vi "Main.vi"() -> ()   [LabVIEW 2020]
uses:
  <vilib>/SAPHIR/GDataBase for MySQL(tm)/MySQL/MySQLConnector.lvclass/MySQLConnector.ctl
  <vilib>/SAPHIR/GDataBase for MySQL(tm)/NetworkStream/MySQLNetworkStream.lvclass/MySQLNetworkStream.ctl
  <vilib>/SAPHIR/GDataBase for MySQL(tm)/NetworkStream/public/SendCommand.vi
  <vilib>/SAPHIR/GDataBase for MySQL(tm)/NetworkStream/public/locker/AcquireLocker.vi
  <vilib>/SAPHIR/GDataBase for MySQL(tm)/NetworkStream/public/locker/ReleaseLocker.vi
  <vilib>/SAPHIR/GDataBase for MySQL(tm)/NetworkStream/public/WritePacket.vi
  <vilib>/Utility/semaphor.llb/Acquire Semaphore.vi
  <vilib>/SAPHIR/GDataBase for MySQL(tm)/NetworkStream/public/ReadResultPacket.vi
  <vilib>/Utility/semaphor.llb/Release Semaphore.vi
  <vilib>/Instr/_visa.llb/VISA Configure Serial Port (Instr).vi
  <vilib>/SAPHIR/GDataBase for MySQL(tm)/MySQL/MySQLConnector.lvclass
panel:
  in  "Stop":bool
  in  "Tab Control":enum32{"Dashboard", "Config"}(tab)
  out "Abanico":bool
  out "Extractor":bool
  out "Presencia de Gas":bool
  out "Alarma de Temperatura":bool
  out "Propano":dbl(slide) scale=0.0..40.0
  out "CO":dbl(slide) scale=0.0..100.0
  out "LPG":dbl(slide) scale=0.0..80.0
  out "Alcohol":dbl(slide) scale=0.0..30.0
  out "H2":dbl(slide) scale=0.0..50.0
  out "Humedad Relativa":dbl(graph)
  out "Temperatura (Celsius)":dbl(graph)
  out "Propano":dbl
  out "CO":dbl
  out "Alcohol":dbl
  out "LPG":dbl
  out "H2":dbl
  out "Hum %":dbl
  out "Temp C":dbl
  out "Fecha":string
  in  "Base de Datos":string
  in  "Password":string
  in  "Usuario":string
  in  "MySQL Server (IP)":string
  in  "Propano":dbl(slide) scale=0.0..100.0
  in  "Alcohol":dbl(slide) scale=0.0..100.0
  in  "CO":dbl(slide) scale=0.0..100.0
  in  "LPG":dbl(slide) scale=0.0..100.0
  in  "H2":dbl(slide) scale=0.0..100.0
  in  "Rango de Temperatura Adecuada":cluster{"Numeric":dbl, "Numeric":dbl}(slide)={"Numeric"=0.0, "Numeric"=6.538461538461539} scale=0.0..50.0
  in  "Puerto Serial":refnum<visa-resource-name>="COM4"
  # "Arduino"
  # "Set Points"
  # "Base de Datos"
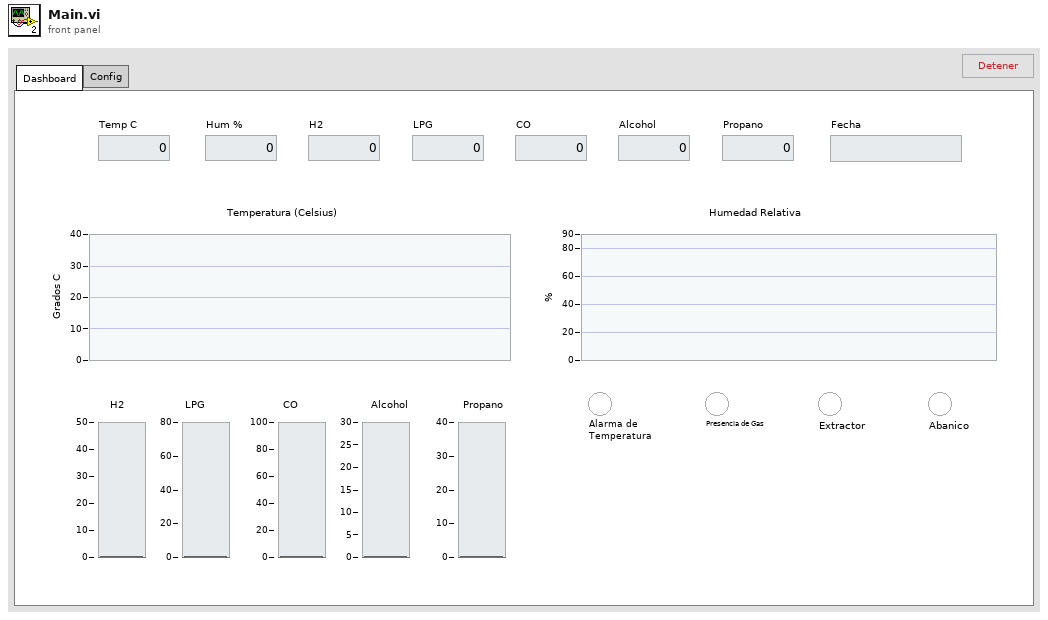
[diagram p1: front panel]
types:
  T1 = cluster{"Usuario":string, "Password":string, "Base de Datos":string}
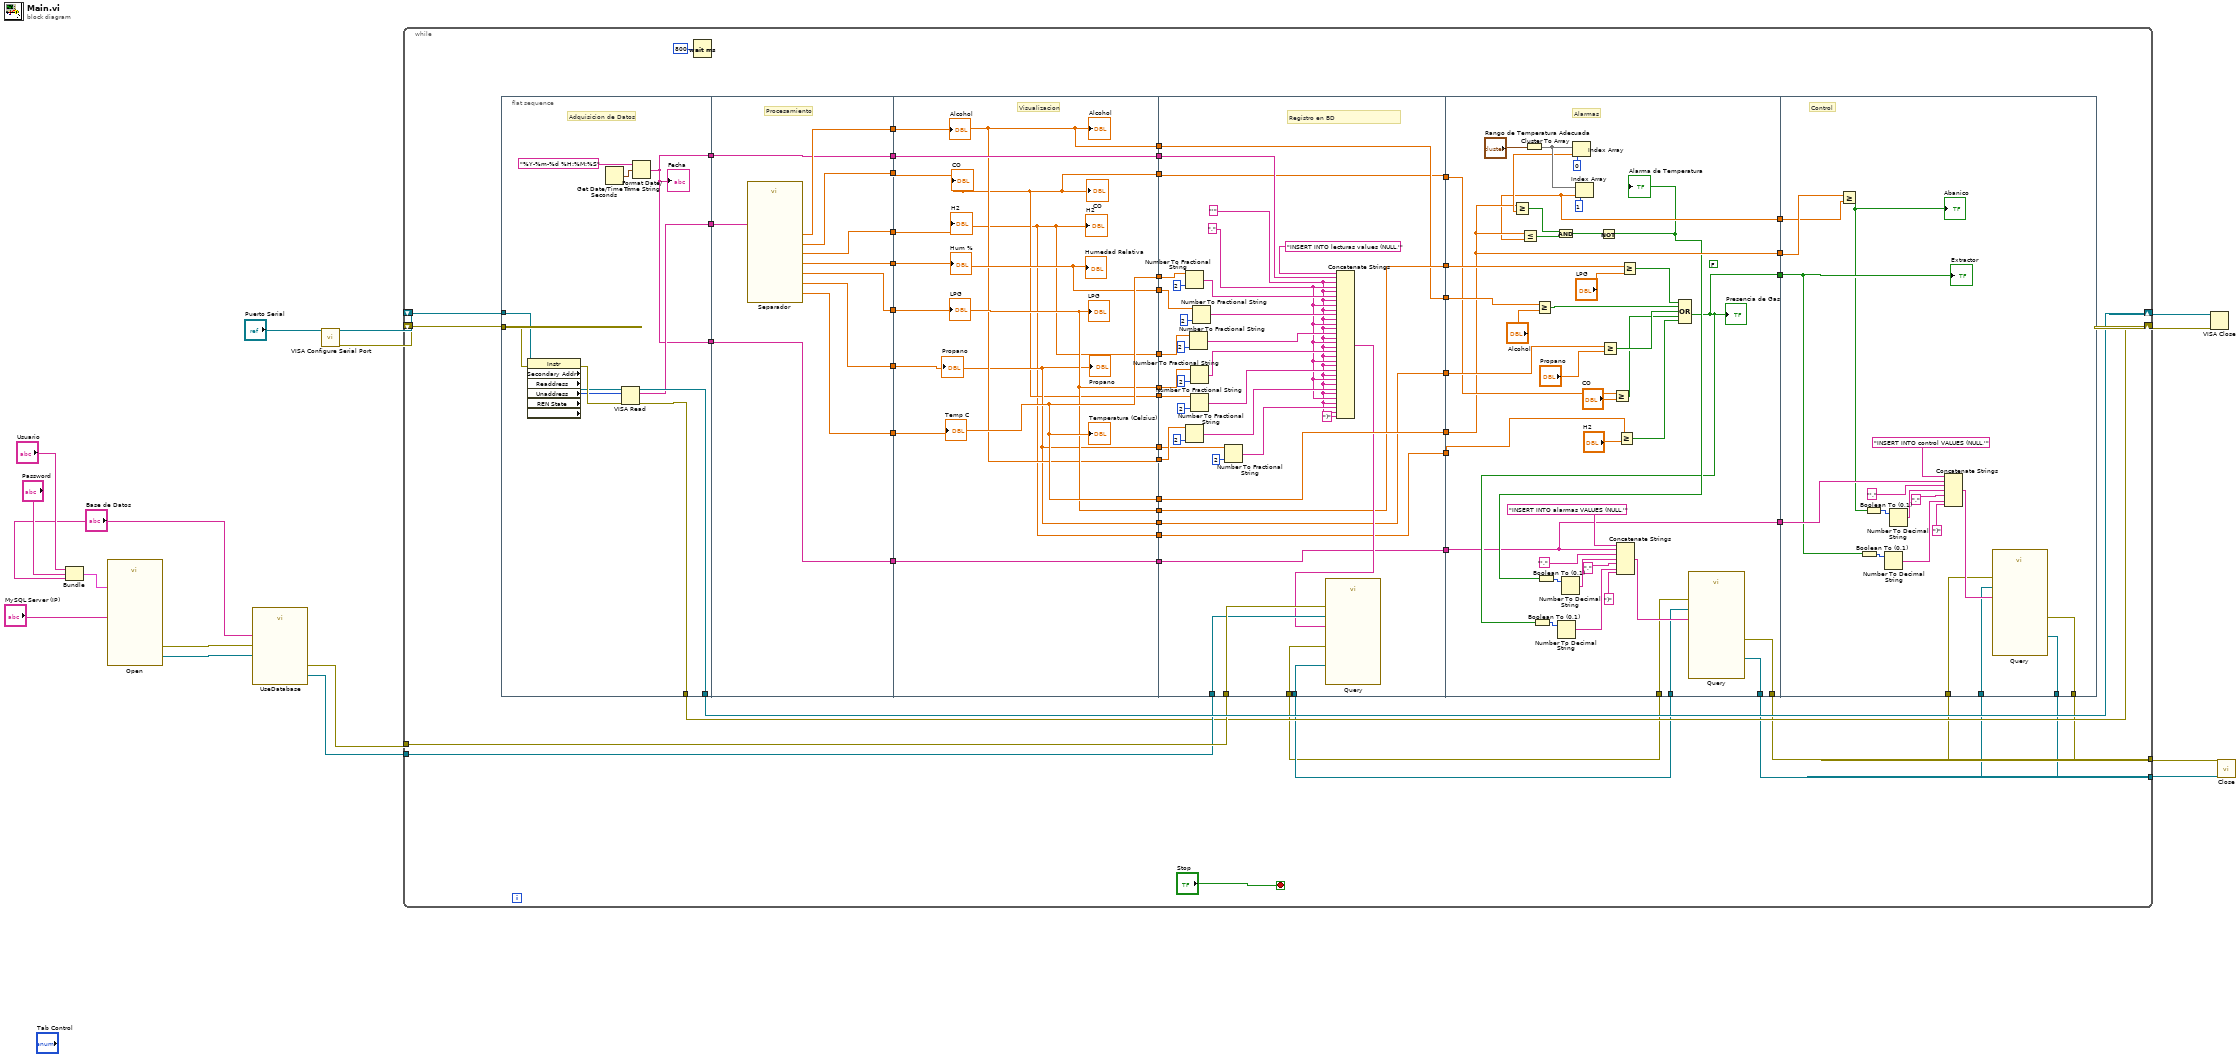
[diagram p0: block diagram]
diagram:
  n1 = Bundle("Usuario"="Usuario", "Password"="Password", "Base de Datos"="Base de Datos") -> (w1:T1)  [unwired: 1 in]
  n2 = call <vilib>:"Open.vi"("clientAuthentication"=w1, "host"="MySQL Server (IP)") -> ("error out"=w15:errorcluster, "MySQL out"=w14:refnum<class "MySQLConnector.lvclass">)  [unwired: 8 in]
  n3 = call <vilib>:"UseDatabase.vi"("error in (no error)"=w15, "databaseName"="Base de Datos", "MySQL in"=w14) -> ("error out"=w7:errorcluster, "MySQL out"=w6:refnum<class "MySQLConnector.lvclass">)  [unwired: 7 in]
  n4 = call-poly "VISA Configure Serial Port"("VISA resource name"="Puerto Serial") -> ("VISA resource name out"=w9:refnum<visa-resource-name>, "error out"=w8:errorcluster)  [unwired: 13 in]
  n5 = while {
    shift-right: [w64] -> w11
    shift-left: w9 -> [w66]
    shift-right: [w24] -> w10
    shift-left: w8 -> [w65]
    tunnel: w7 -> [w53]
    tunnel: w6 -> [w52]
    tunnel: [w19] -> w12
    tunnel: [w17] -> w13
    stop <- "Stop" stop-if-true
    n6 = flat-sequence {
      tunnel: w66 -> [w79]
      tunnel: w65 -> [w78]
      tunnel: [w74] -> w24
      tunnel: [w73] -> w64
      tunnel: [w72] -> w56
      tunnel: [w69] -> w49
      tunnel: [w69] -> w28
      tunnel: [w89] -> w63
      tunnel: [w88] -> w62
      tunnel: [w87] -> w61
      tunnel: [w86] -> w60
      tunnel: [w85] -> w59
      tunnel: [w84] -> w58
      tunnel: [w83] -> w57
      tunnel: w56 -> [w82]
      tunnel: [w81] -> w50
      tunnel: w49 -> [w81]
      tunnel: w28 -> [w80]
      tunnel: [w80] -> w27
      tunnel: w63 -> [w94]
      tunnel: w62 -> [w92]
      tunnel: w61 -> [w91]
      tunnel: w60 -> [w96]
      tunnel: w59 -> [w95]
      tunnel: w58 -> [w93]
      tunnel: w57 -> [w97]
      tunnel: [w97] -> w55
      tunnel: [w98] -> w51
      tunnel: w50 -> [w98]
      tunnel: [w97] -> w48
      tunnel: [w96] -> w47
      tunnel: [w91] -> w46
      tunnel: [w95] -> w45
      tunnel: [w92] -> w44
      tunnel: [w94] -> w43
      tunnel: [w93] -> w42
      tunnel: [w95] -> w41
      tunnel: [w94] -> w39
      tunnel: [w93] -> w37
      tunnel: [w92] -> w34
      tunnel: [w91] -> w33
      tunnel: w27 -> [w90]
      tunnel: [w90] -> w26
      tunnel: w55 -> [w136]
      tunnel: [w136] -> w54
      tunnel: w53 -> [w135]
      tunnel: w52 -> [w134]
      tunnel: [w133] -> w22
      tunnel: [w132] -> w23
      tunnel: w51 -> [w130]
      tunnel: w48 -> [w129]
      tunnel: w47 -> [w127]
      tunnel: w46 -> [w125]
      tunnel: w45 -> [w120]
      tunnel: w44 -> [w116]
      tunnel: w43 -> [w112]
      tunnel: w42 -> [w106]
      tunnel: w41 -> [w104]
      tunnel: [w104] -> w40
      tunnel: w39 -> [w103]
      tunnel: [w103] -> w38
      tunnel: w37 -> [w102]
      tunnel: [w102] -> w36
      tunnel: [w101] -> w35
      tunnel: w34 -> [w101]
      tunnel: w33 -> [w100]
      tunnel: [w100] -> w32
      tunnel: w26 -> [w99]
      tunnel: [w99] -> w25
      tunnel: w54 -> [w154]
      tunnel: w40 -> [w165]
      tunnel: w38 -> [w164]
      tunnel: w36 -> [w163]
      tunnel: w35 -> [w162]
      tunnel: w32 -> [w161]
      tunnel: [w142] -> w31
      tunnel: [w154] -> w30
      tunnel: [w153] -> w29
      tunnel: w25 -> [w137]
      tunnel: w23 -> [w146]
      tunnel: w22 -> [w145]
      tunnel: [w144] -> w18
      tunnel: [w143] -> w20
      tunnel: [w137] -> w21
      tunnel: w31 -> [w183]
      tunnel: w30 -> [w195]
      tunnel: w29 -> [w194]
      tunnel: w21 -> [w184]
      tunnel: w20 -> [w181]
      tunnel: w18 -> [w180]
      tunnel: [w179] -> w19
      tunnel: [w178] -> w17
      frame #0 {
        # "Adquisicion de Datos"
        n7 = property class="Instr" props=["Secondary Addr", "Readdress", "Unaddress", "REN State", "Serial Settings:Number of Bytes at Serial Port"](reference=w79, error in=w78) -> (reference out=w75:refnum<visa-resource-name>, error out=w77:errorcluster, "Serial Settings:Number of Bytes at Serial Port"=w76:u32)  [unwired: 4 out]
        n8 = Get Date/Time In Seconds() -> (seconds since 1Jan1904=w71:timestamp)
        n9 = VISA Read(VISA resource name=w75, byte count=w76, error in (no error)=w77) -> (VISA resource name out=w73:refnum<visa-resource-name>, read buffer=w72:string, error out=w74:errorcluster)  [unwired: 1 out]
        n10 = Format Date/Time String(time format string (%c)="%Y-%m-%d %H:%M:%S", seconds (now)=w71) -> (date/time string=w69:string)  [unwired: 1 in]
        "Fecha" <- w69
      }
      frame #1 {
        # "Procesamiento"
        n11 = call "Separador.vi"("Lectura del puerto Serial"=w82) -> ("Propano"=w84:dbl, "ALcohol"=w89:dbl, "CO"=w88:dbl, "LPG"=w85:dbl, "H2"=w87:dbl, "Humedad"=w86:dbl, "Temperatura"=w83:dbl)
      }
      frame #2 {
        # "Visualizacion"
        "Alcohol" <- w94
        "CO" <- w92
        "H2" <- w91
        "LPG" <- w95
        "Propano" <- w93
        "Temp C" <- w97
        "Hum %" <- w96
        "Temperatura (Celsius)" <- w97
        "Humedad Relativa" <- w96
        "H2" <- w91
        "Alcohol" <- w94
        "Propano" <- w93
        "CO" <- w92
        "LPG" <- w95
      }
      frame #3 {
        w110 = ","
        w108 = "'"
        # "Registro en BD"
        n12 = Number To Fractional String(number=w129, precision (6)=i16 2) -> (F-format string=w128:string)  [unwired: 2 in]
        n13 = Number To Fractional String(number=w112, precision (6)=i16 2) -> (F-format string=w111:string)  [unwired: 2 in]
        n14 = Number To Fractional String(number=w125, precision (6)=i16 2) -> (F-format string=w124:string)  [unwired: 2 in]
        n15 = Number To Fractional String(number=w120, precision (6)=i16 2) -> (F-format string=w118:string)  [unwired: 2 in]
        n16 = Number To Fractional String(number=w116, precision (6)=i16 2) -> (F-format string=w117:string)  [unwired: 2 in]
        n17 = Number To Fractional String(number=w127, precision (6)=i16 2) -> (F-format string=w126:string)  [unwired: 2 in]
        n18 = Number To Fractional String(number=w106, precision (6)=i16 2) -> (F-format string=w109:string)  [unwired: 2 in]
        n19 = Concatenate Strings("INSERT INTO lecturas values (NULL,'" ("string"), w130, w108, w110, w108, w128, w108, w110, w108, w126, w108, w110, w108, w124, w108, w110, w108, w118, w108, w110, w108, w117, w108, w110, w108, w111, w108, w110, w108, w109, w108, ")" ("string")) -> (w105:string)
        n20 = call <vilib>:"Query.vi"("error in (no error)"=w135, "query"=w105, "MySQL in"=w134) -> ("error out"=w133:errorcluster, "MySQL out"=w132:refnum<class "MySQLConnector.lvclass">)  [unwired: 5 in, 2 out]
      }
      frame #4 {
        (unwired) FALSE (".not. x?")
        # "Alarmas"
        n21 = Cluster To Array(cluster="Rango de Temperatura Adecuada") -> (array=w177:dbl[])
        n22 = Greater Or Equal?(x=w164, y="Alcohol") -> (x >= y?=w159:bool)
        n23 = Index Array(array=w177, index=0) -> (element=w173:dbl)
        n24 = Greater Or Equal?(x=w154, y=w173) -> (x >= y?=w155:bool)
        n25 = Index Array(array=w177, index=1) -> (element=w153:dbl)
        n26 = Less Or Equal?(x=w154, y=w153) -> (x <= y?=w172:bool)
        n27 = And(x=w155, y=w172) -> (x .and. y?=w171:bool)
        n28 = Not(x=w171) -> (.not. x?=w150:bool)
        "Alarma de Temperatura" <- w150
        n29 = Boolean To (0,1)(Boolean=w150) -> (0, 1=w149:i16)
        n30 = Number To Decimal String(number=w149) -> (decimal integer string=w148:string)  [unwired: 1 in]
        n31 = Greater Or Equal?(x=w163, y="Propano") -> (x >= y?=w158:bool)
        n32 = Greater Or Equal?(x=w162, y="CO") -> (x >= y?=w157:bool)
        n33 = Greater Or Equal?(x=w161, y="H2") -> (x >= y?=w156:bool)
        n34 = Greater Or Equal?(x=w165, y="LPG") -> (x >= y?=w160:bool)
        n35 = Compound Arithmetic op=OR(w160, w159, w158, w157, w156) -> (w142:bool)
        "Presencia de Gas" <- w142
        n36 = Boolean To (0,1)(Boolean=w142) -> (0, 1=w141:i16)
        n37 = Number To Decimal String(number=w141) -> (decimal integer string=w139:string)  [unwired: 1 in]
        n38 = Concatenate Strings("INSERT INTO alarmas VALUES (NULL,'", w137, "'," ("string"), w148, "," ("string"), w139, ")" ("string")) -> (w147:string)
        n39 = call <vilib>:"Query.vi"("error in (no error)"=w145, "query"=w147, "MySQL in"=w146) -> ("error out"=w143:errorcluster, "MySQL out"=w144:refnum<class "MySQLConnector.lvclass">)  [unwired: 5 in, 2 out]
      }
      frame #5 {
        # "Control"
        n40 = Greater Or Equal?(x=w195, y=w194) -> (x >= y?=w182:bool)
        "Abanico" <- w182
        n41 = Boolean To (0,1)(Boolean=w183) -> (0, 1=w189:i16)
        n42 = Boolean To (0,1)(Boolean=w182) -> (0, 1=w191:i16)
        n43 = Number To Decimal String(number=w189) -> (decimal integer string=w187:string)  [unwired: 1 in]
        n44 = Number To Decimal String(number=w191) -> (decimal integer string=w190:string)  [unwired: 1 in]
        n45 = Concatenate Strings("INSERT INTO control VALUES (NULL,'", w184, "'," ("string"), w190, "," ("string"), w187, ")" ("string")) -> (w185:string)
        n46 = call <vilib>:"Query.vi"("error in (no error)"=w181, "query"=w185, "MySQL in"=w180) -> ("error out"=w179:errorcluster, "MySQL out"=w178:refnum<class "MySQLConnector.lvclass">)  [unwired: 5 in, 2 out]
        "Extractor" <- w183
      }
    }
    n47 = Wait (ms)(milliseconds to wait=u32 800) -> ()  [unwired: 1 out]
  }
  n48 = VISA Close(VISA resource name=w11, error in (no error)=w10) -> ()  [unwired: 1 out]
  n49 = call <vilib>:"Close.vi"("error in (no error)"=w12, "MySQL in"=w13) -> ()  [unwired: 9 in, 1 out]
